vi "Acquisition.vi"(0 "connection ID":refnum<k5>, 1 "ACQ stop by events":T1={"ACQ stop by events button"=FALSE, "Events to acquire"=1000} caption="Stop by events" {"Events to acquire" min=1}, 2 "ACQ parameters":u32[](array[numeric])=[0, 0, 0, 0], 3 "File ACQ data":path=path "C:/VIP Module/Files/ACQbinaryData.dat", 4 "LayerID":u32=65535 format="%x", 5 "ChipID":u32=65535 format="%x", 6 "Stop ACQ button Refnum":refnum<vi>, 7 "error in (no error)":errorcluster, 8 "ACQ barra Refnum":refnum<vi>, 10 "Actual time Refnum":refnum<vi>, 12 "Acquisition time Refnum":refnum<vi>, 16 "Events Refnum":refnum<vi>) -> (13 "Stop by events":bool, 15 "ACQ WatchDog timeout":bool, 17 "Answer":string, 20 "connection ID out":refnum<k5>, 25 "error out comm":errorcluster, 27 "error out file":errorcluster)   [LabVIEW 2015, in "VIPM2.lvlib"]
uses:
  VIPM2.lvlib
panel:
  out "Ready to receive parameters":string
  # "Acquisition in progress..."
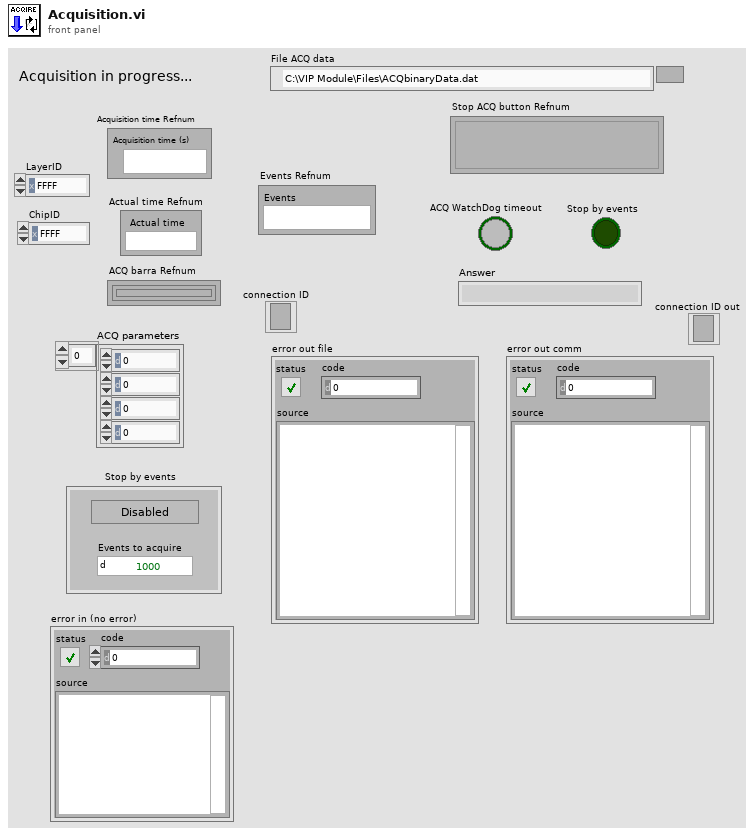
[diagram p1: front panel]
types:
  T1 = cluster{"ACQ stop by events button":bool, "Events to acquire":u32}
  T2 = enum16{"open", "replace", "create", "open or create", "replace or create", "replace or create with confirmation"}
  T3 = enum16{"Standard", "Buffered", "CRLF", "Immediate"}
  T4 = enum16{"big-endian, network order", "native, host order", "little-endian"}
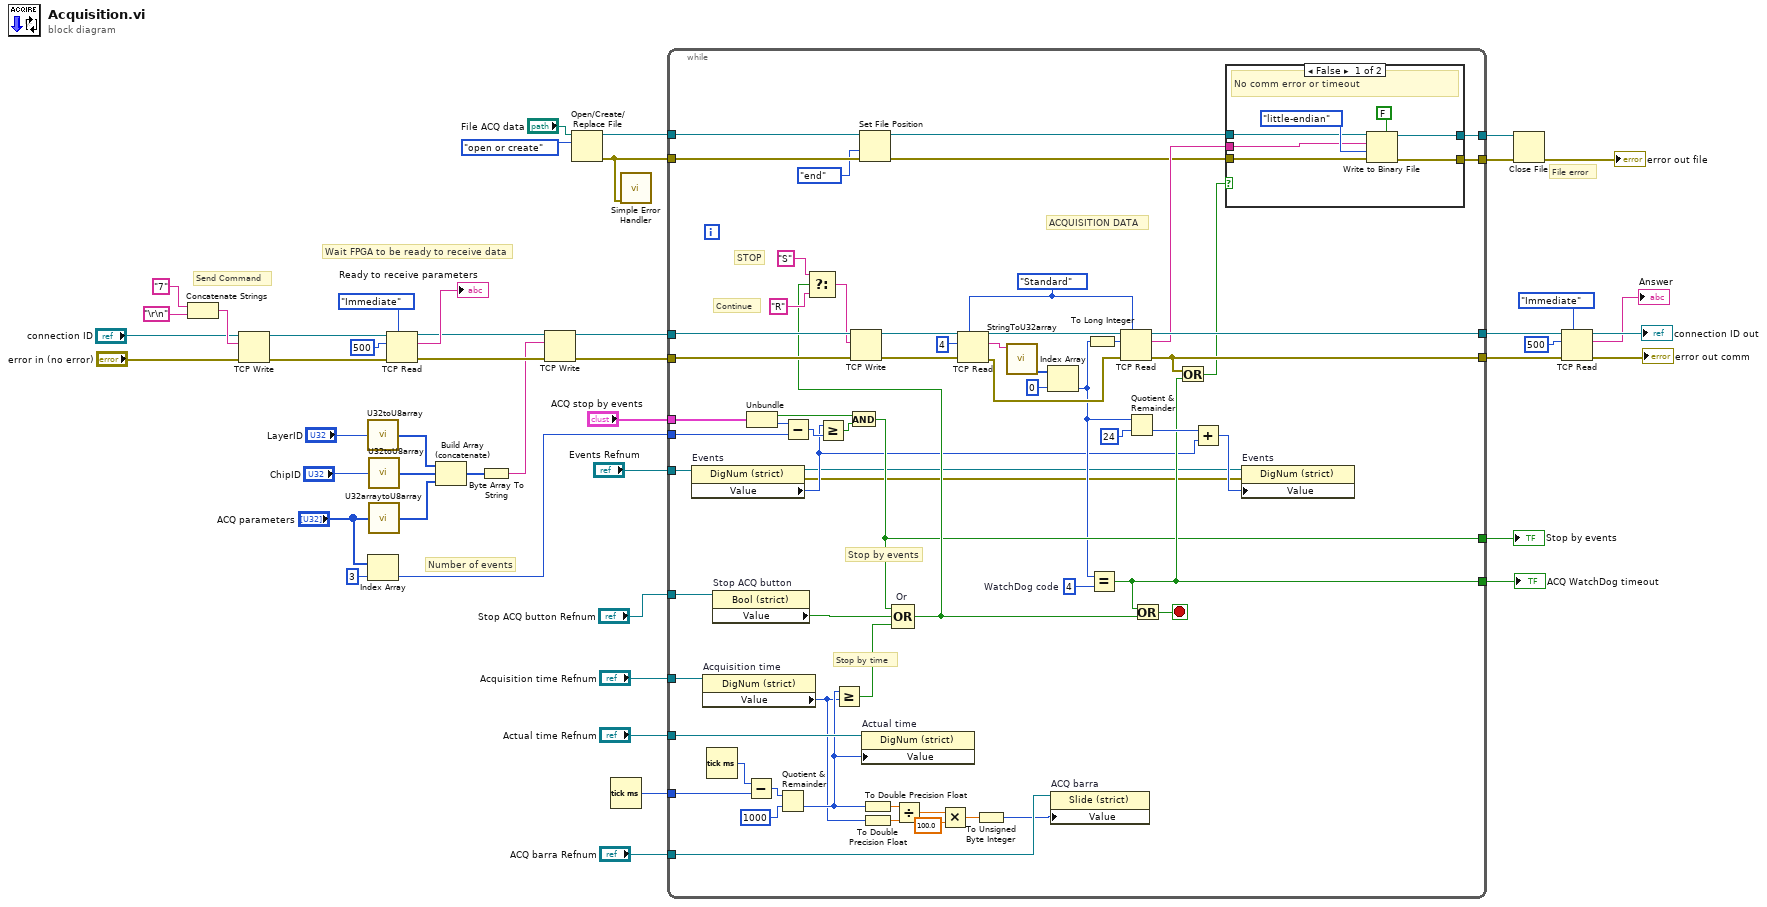
[diagram p0: block diagram]
diagram:
  # "Number of events"
  # "File error"
  # "Wait FPGA to be ready to receive data"
  # "Send Command"
  n1 = Concatenate Strings("7" ("string"), "\r\n") -> (w45:string)
  n2 = TCP Write(connection ID="connection ID", data in=w45, error in (no error)="error in (no error)") -> (connection ID out=w39:refnum<k5>, error out=w38:errorcluster)  [unwired: 1 in, 1 out]
  n3 = call "U32toU8array.vi"("x"="LayerID") -> ("ArrayU8"=w28:u8[])
  n4 = Index Array "Index Array"(array="ACQ parameters", index=3) -> (element=w9:u32)
  n5 = call "U32toU8array.vi"("x"="ChipID") -> ("ArrayU8"=w26:u8[])
  n6 = call "U32arraytoU8array.vi"("ArrayU32"="ACQ parameters") -> ("ArrayU8"=w25:u8[])
  n7 = TCP Read(connection ID=w39, bytes to read=500, error in (no error)=w38, 7:T3."Immediate" ("mode (standard)")) -> (connection ID out=w36:refnum<k5>, data out=→"Ready to receive parameters":string, error out=w35:errorcluster)  [unwired: 1 in]
  n8 = Build Array (concatenate)(w28, w26, w25) -> (w29:u8[])
  n9 = Byte Array To String(unsigned byte array=w29) -> (string=w34:string)
  n10 = TCP Write(connection ID=w36, data in=w34, error in (no error)=w35) -> (connection ID out=w24:refnum<k5>, error out=w23:errorcluster)  [unwired: 1 in, 1 out]
  n11 = Open/Create/Replace File(file path (use dialog)="File ACQ data", operation (0:open)=T2."open or create") -> (refnum out=w20:refnum<file>, error out=w14:errorcluster)  [unwired: 4 in, 1 out]
  n12 = Tick Count (ms)() -> (millisecond timer value=w15:u32)
  n13 = call <vilib>:"Simple Error Handler.vi"("error in (no error)"=w14) -> ()  [unwired: 4 in, 5 out]
  n14 = while {
    tunnel: w24 -> [w108]
    tunnel: w23 -> [w107]
    tunnel: w14 -> [w84]
    tunnel: w20 -> [w85]
    tunnel: [w79] -> w19
    tunnel: [w95] -> w18
    tunnel: [w94] -> w17
    tunnel: [w93] -> w16
    tunnel: w15 -> [w90]
    tunnel: w9 -> [w73]
    tunnel: [w69] -> w8
    tunnel: "Acquisition time Refnum" -> [w66]
    tunnel: [w68] -> w7
    tunnel: "ACQ stop by events" -> [w67]
    tunnel: "Actual time Refnum" -> [w65]
    tunnel: "ACQ barra Refnum" -> [w57]
    tunnel: "Events Refnum" -> [w54]
    tunnel: "Stop ACQ button Refnum" -> [w49]
    stop <- w92 stop-if-true
    w100 = u32 4  # WatchDog code
    w103 = T3."Standard" ("mode (standard)")
    # "Stop by events"
    # "Stop by time"
    # "ACQUISITION DATA"
    # "Continue"
    # "STOP"
    n15 = property on="Events" class="DigNum (strict)"(reference=w54) -> (reference out=w51:refnum<vi>, error out=w50:errorcluster, "Value"=w53:u32)  [unwired: 1 in]
    n16 = property on="Acquisition time" class="DigNum (strict)"(reference=w66) -> ("Value"=w58:u32)  [unwired: 1 in, 2 out]
    n17 = Tick Count (ms)() -> (millisecond timer value=w91:u32)
    n18 = property on="Stop ACQ button" class="Bool (strict)"(reference=w49) -> ("Value"=w48:bool)  [unwired: 1 in, 2 out]
    n19 = Subtract(x=w91, y=w90) -> (x-y=w87:u32)
    n20 = Unbundle(w67) -> ("ACQ stop by events button"=w74:bool, "Events to acquire"=w71:u32)
    n21 = Quotient & Remainder(x=w87, y=u32 1000) -> (floor(x/y)=w59:u32)  [unwired: 1 out]
    n22 = Subtract(x=w71, y=w73) -> (x-y=w70:u32)
    n23 = Greater Or Equal?(x=w53, y=w70) -> (x >= y?=w72:bool)
    n24 = Greater Or Equal?(x=w59, y=w58) -> (x >= y?=w89:bool)
    n25 = And(x=w74, y=w72) -> (x .and. y?=w68:bool)
    n26 = Set File Position(refnum=w85, from (0:start)=enum16{"start", "end", "current"}."end", error in=w84) -> (refnum out=w80:refnum<file>, error out=w81:errorcluster)  [unwired: 1 in]
    n27 = property on="Actual time" class="DigNum (strict)"(reference=w65, "Value"=w59) -> ()  [unwired: 1 in, 2 out]
    n28 = To Double Precision Float(number=w59) -> (double precision float=w61:dbl)
    n29 = To Double Precision Float(number=w58) -> (double precision float=w60:dbl)
    n30 = Compound Arithmetic op=OR "Or"(w68, w48, w89) -> (w88:bool)
    n31 = Select(t="S" ("string"), s=w88, f="R" ("string")) -> (s? t:f=w106:string)
    n32 = TCP Write(connection ID=w108, data in=w106, error in (no error)=w107) -> (connection ID out=w99:refnum<k5>, error out=w98:errorcluster)  [unwired: 1 in, 1 out]
    n33 = Divide(x=w61, y=w60) -> (x/y=w62:dbl)
    n34 = Multiply(x=w62, y=100.0) -> (x*y=w64:dbl)
    n35 = TCP Read(connection ID=w99, bytes to read=4, error in (no error)=w98, 7:w103) -> (connection ID out=w101:refnum<k5>, data out=w97:string, error out=w102:errorcluster)  [unwired: 1 in]
    n36 = To Unsigned Byte Integer(number=w64) -> (unsigned 8bit integer=w56:u8)
    n37 = call "StringToU32array.vi"("String"=w97) -> ("U32array"=w96:u32[])  [unwired: 2 out]
    n38 = Index Array(array=w96, index=0) -> (element=w55:u32)
    n39 = property on="ACQ barra" class="Slide (strict)"(reference=w57, "Value"=w56) -> ()  [unwired: 1 in, 2 out]
    n40 = To Long Integer(number=w55) -> (32bit integer=w75:i32)
    n41 = Equal?(x=w55, y=w100) -> (x = y?=w69:bool)
    n42 = TCP Read(connection ID=w101, bytes to read=w75, error in (no error)=w102, 7:w103) -> (connection ID out=w95:refnum<k5>, data out=w82:string, error out=w79:errorcluster)  [unwired: 1 in]
    n43 = Quotient & Remainder(x=w55, y=u32 24) -> (floor(x/y)=w77:u32)  [unwired: 1 out]
    n44 = Or(x=w69, y=w88) -> (x .or. y?=w92:bool)
    n45 = Or(x=w79, y=w69) -> (x .or. y?=w78:bool)
    n46 = Add(x=w77, y=w53) -> (x+y=w52:u32)
    n47 = case shown="False" w78 {
      tunnel: [w115 w119] -> w94
      tunnel: [w114 w118] -> w93
      tunnel: w82 -> [w113 _]
      tunnel: w81 -> [w112 w118]
      tunnel: w80 -> [w111 w119]
      frame False {
        # "No comm error or timeout"
        n48 = Write to Binary File(file (use dialog)=w111, data=w113, error in=w112, 5:FALSE ("prepend array or string size? (T)"), 9:T4."little-endian" ("byte order (0:big-endian, network order)")) -> (refnum out=w115:refnum<file>, error out=w114:errorcluster)  [unwired: 1 in, 1 out]
      }
      frame True {
      }
    }
    n49 = property on="Events" class="DigNum (strict)"(reference=w51, error in=w50, "Value"=w52) -> ()  [unwired: 2 out]
  }
  "ACQ WatchDog timeout" <- w8
  "Stop by events" <- w7
  n50 = Close File(refnum=w17, error in=w16) -> (error out=→"error out file":errorcluster)  [unwired: 1 out]
  n51 = TCP Read(connection ID=w18, bytes to read=500, error in (no error)=w19, 7:T3."Immediate" ("mode (standard)")) -> (connection ID out=→"connection ID out":refnum<k5>, data out=→"Answer":string, error out=→"error out comm":errorcluster)  [unwired: 1 in]
